vi "CMD_SUM (SubVI).vi"(1 "value":string, 2 "Func":string) -> (0 "String":string)   [LabVIEW 8.6]
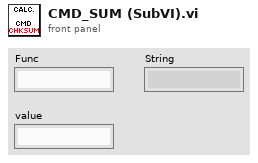
[diagram p1: front panel]
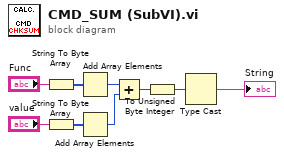
[diagram p0: block diagram]
diagram:
  n1 = String To Byte Array(string="Func") -> (unsigned byte array=w1:u8[])
  n2 = String To Byte Array(string="value") -> (unsigned byte array=w3:u8[])
  n3 = Add Array Elements(numeric array=w1) -> (sum=w5:u8)
  n4 = Add Array Elements(numeric array=w3) -> (sum=w4:u8)
  n5 = Add(x=w5, y=w4) -> (x+y=w7:u8)
  n6 = To Unsigned Byte Integer(number=w7) -> (unsigned 8bit integer=w8:u8)
  n7 = Type Cast(x=w8) -> (*(type *) &x=→"String":string)  [unwired: 1 in]
